vi "Set Virtual Instr Configuration.vi"(8 "error in (no error)":errorcluster, 10 "Virt Instr CFG":string, 11 "Configuration UI Actor in":refnum<class "Configuration UI Actor.lvclass">) -> (0 "error out":errorcluster, 3 "Configuration UI Actor out":refnum<class "Configuration UI Actor.lvclass">)   [LabVIEW 2023, in "Configuration UI Actor.lvlib" / "Configuration UI Actor.lvclass"]
uses:
  Configuration UI Actor.lvclass
  Configuration UI Actor.lvclass/Configuration UI Actor.ctl
  <vilib>/JDP Science/JSONtext/JSONtext.lvlib
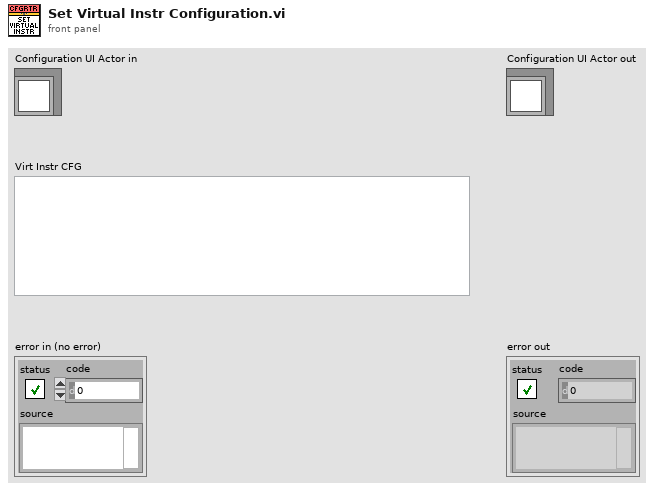
[diagram p1: front panel]
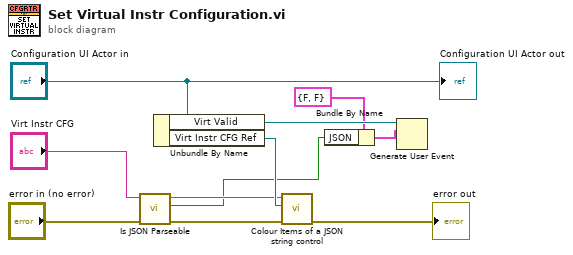
[diagram p0: block diagram]
diagram:
  n1 = call "Is JSON Parseable.vi"("error in (no error)"="error in (no error)", "<JSON>"="Virt Instr CFG") -> ("error out"=w5:errorcluster, "Valid?"=w1:bool, "Pretty <JSON>"=w6:string)  [unwired: 7 in]
  n2 = Unbundle By Name("Configuration UI Actor in") -> ("Virt Valid"=w4:refnum<user-event>, "Virt Instr CFG Ref"=w9:refnum<vi>)
  n3 = call <vilib>:"Colour Items of a JSON string control.vi"("error in (no error)"=w5, "String Control"=w9, "JSON"=w6) -> ("error out"=→"error out":errorcluster)  [unwired: 8 in]
  n4 = Bundle By Name(cluster=cluster{"JSON":bool, "CFG":bool} {"JSON"=FALSE, "CFG"=FALSE} ("Virt Valid"), "JSON"=w1) -> (w2:cluster{"JSON":bool, "CFG":bool})
  n5 = Generate User Event(user event=w4, event data cluster=w2) -> ()  [unwired: 2 in, 2 out]
  "Configuration UI Actor out" <- "Configuration UI Actor in"
